vi "saveDataNodeBegin.vi"(8 "error in (no error)":errorcluster, 9 "indent":i32, 10 "XML Refnum in":refnum<file>, 11 "PWM in":refnum<class "PWM.lvclass">) -> (0 "error out":errorcluster, 2 "XML Refnum out":refnum<file>, 3 "PWM out":refnum<class "PWM.lvclass">)   [LabVIEW 2013, in "PWM.lvclass"]
doc: "Begins the process of saving a xceData Node to an XML formatted file."
uses:
  PWM.lvclass
  Channel/Channel.lvclass
  xCE/xceNode/xceNode.lvclass
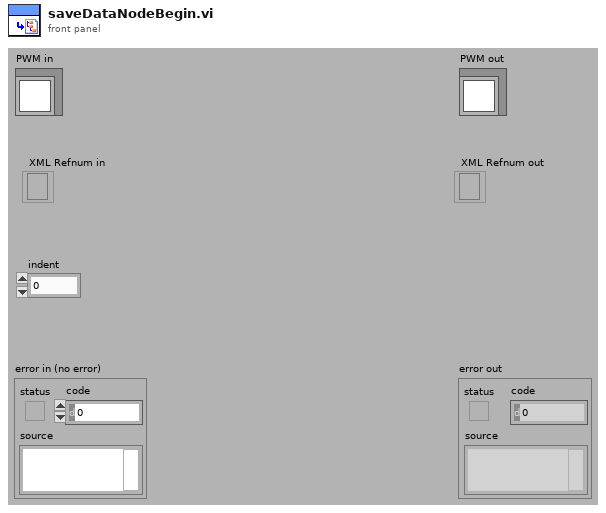
[diagram p1: front panel]
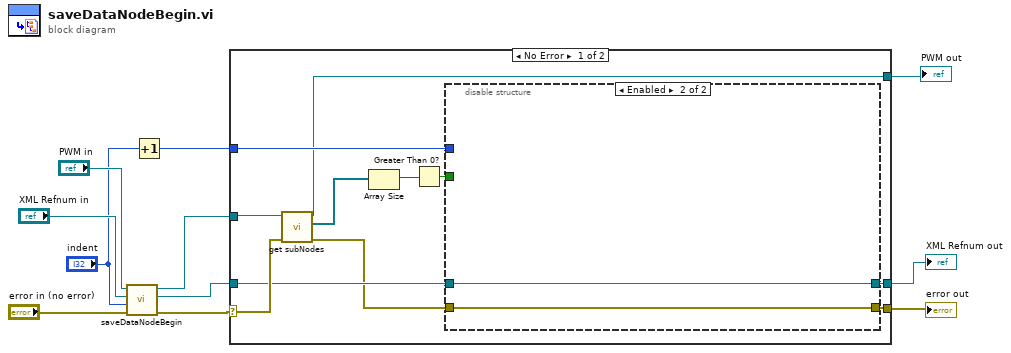
[diagram p0: block diagram]
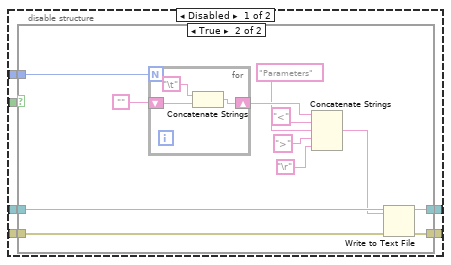
[diagram p2: hidden frame]
diagram:
  n1 = call-parent "saveDataNodeBegin.vi"("error in (no error)"="error in (no error)", "indent"="indent", "XML Refnum in"="XML Refnum in", "Channel in"="PWM in") -> ("error out"=w7:errorcluster, "XML Refnum out"=w6:refnum<file>, "Chennel out"=w8:refnum<class "PWM.lvclass">)  [unwired: 5 in]
  n2 = Increment(x="indent") -> (x+1=w1:i32)
  n3 = case shown="No Error" w7 {
    selector: w7 -> [w22 w48]
    tunnel: w8 -> [w21 w50]
    tunnel: w1 -> [w13 _]
    tunnel: w6 -> [w17 w49]
    tunnel: [w14 w49] -> w4
    tunnel: [w12 w50] -> w3
    tunnel: [w15 w48] -> w5
    frame No Error {
      n4 = call "get subNodes.vi"("error in (no error)"=w22, "xceNode in"=w21) -> ("error out"=w16:errorcluster, "subNodes[]*"=w20:refnum<data-value>[], "xceNode out"=w12:refnum<class "PWM.lvclass">)  [unwired: 7 in]
      n5 = Array Size(array=w20) -> (size(s)=w19:i32)
      n6 = Greater Than 0?(x=w19) -> (x > 0?=w18:bool)
      n7 = disable-structure shown="Enabled" {
        disable-tunnel: w18 -> [w28 _]
        disable-tunnel: w17 -> [w27 w47]
        disable-tunnel: w16 -> [w26 w46]
        disable-tunnel: [w25 w46] -> w15
        disable-tunnel: [w24 w47] -> w14
        disable-tunnel: w13 -> [w23 _]
        frame Disabled {
          n8 = case shown="True" w28 {
            tunnel: w23 -> [_ w37]
            tunnel: w27 -> [w30 w35]
            tunnel: w26 -> [w29 w33]
            tunnel: [w29 w32] -> w25
            tunnel: [w30 w31] -> w24
            frame False {
            }
            frame True {
              n9 = for {
                N: w37 -> [_]
                shift-right: [w45] -> w38
                shift-left: "" -> [w44]
                n10 = Concatenate Strings("\t", w44) -> (w45:string)
              }
              n11 = Concatenate Strings(w38, "<", "Parameters" ("string"), ">", "\r") -> (w34:string)
              n12 = Write to Text File(file (use dialog)=w35, text=w34, error in=w33) -> (refnum out=w31:refnum<file>, error out=w32:errorcluster)  [unwired: 1 in, 1 out]
            }
          }
        }
        frame Enabled {
        }
      }
    }
    frame Error {
    }
  }
  "error out" <- w5
  "PWM out" <- w3
  "XML Refnum out" <- w4
